vi "ReleaseQueue.vi"(8 "error in (no error)":errorcluster, 11 "QueueIN":refnum<queue>) -> (0 "error out":errorcluster)   [LabVIEW 2018]
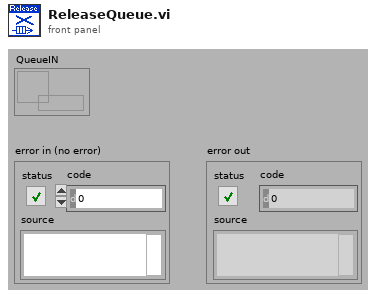
[diagram p1: front panel]
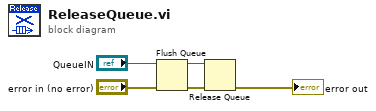
[diagram p0: block diagram]
diagram:
  n1 = Flush Queue(queue="QueueIN", error in (no error)="error in (no error)") -> (queue out=w5:refnum<queue>, error out=w4:errorcluster)  [unwired: 1 out]
  n2 = Release Queue(queue=w5, error in (no error)=w4) -> (error out=→"error out":errorcluster)  [unwired: 3 out]
